vi "sort-sce-list.vi"(11 "模式列表":T1(array[cluster]) {"sce-pannel-list"."pannel"."ID" format="%02x"}) -> (3 "模式列表-sorted":T1(array[cluster]))   [LabVIEW 2019]
panel:
  in  "模式列表 4":T1(array[cluster]) {"sce-pannel-list"."pannel"."ID" format="%02x"}
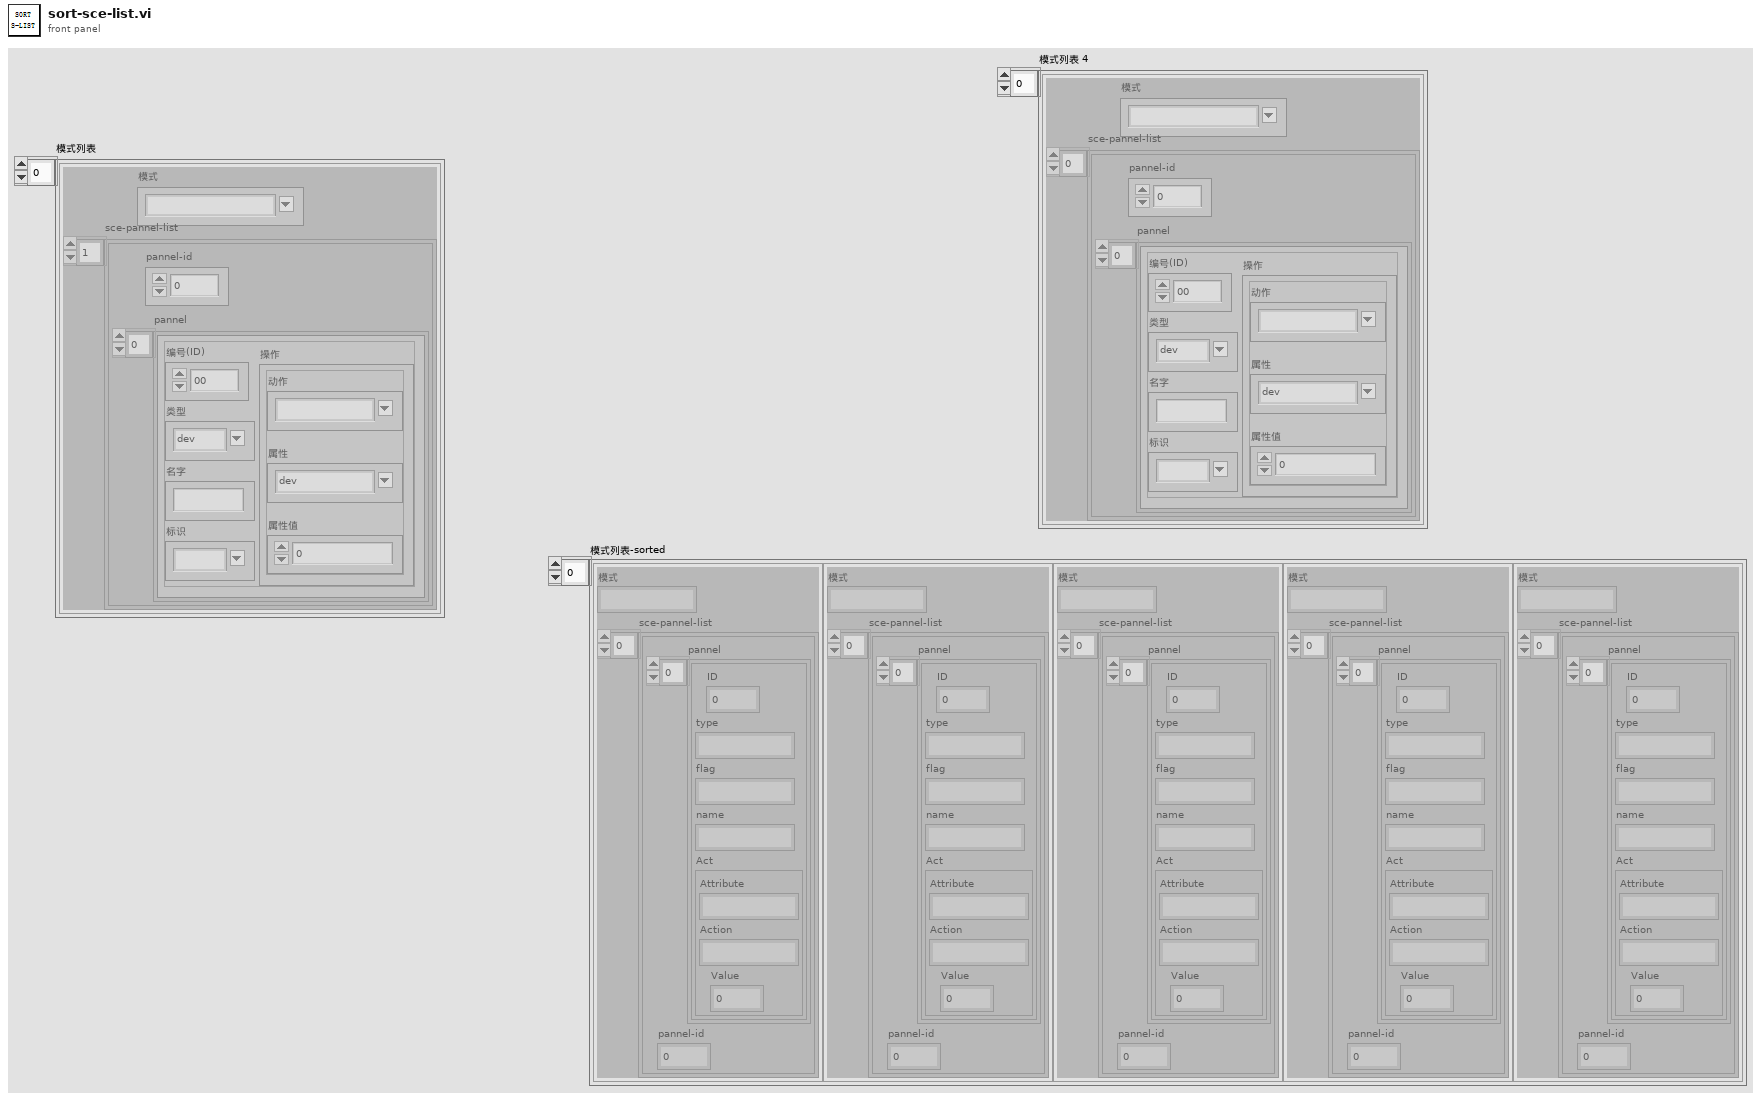
[diagram p1: front panel]
types:
  T1 = cluster{"模式":string, "sce-pannel-list":cluster{"pannel":cluster{"ID":u8, "type":string, "flag":string, "name":string, "Act":cluster{"Attribute":string, "Action":string, "Value":dbl}}[], "pannel-id":dbl}[]}[]
  T2 = cluster{"模式":string, "sce-pannel-list":cluster{"pannel":cluster{"ID":u8, "type":string, "flag":string, "name":string, "Act":cluster{"Attribute":string, "Action":string, "Value":dbl}}[], "pannel-id":dbl}[]}
  T3 = cluster{"pannel":cluster{"ID":u8, "type":string, "flag":string, "name":string, "Act":cluster{"Attribute":string, "Action":string, "Value":dbl}}[], "pannel-id":dbl}[]
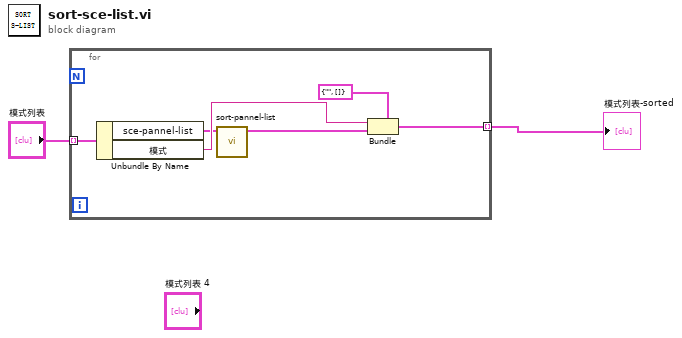
[diagram p0: block diagram]
diagram:
  n1 = for {
    tunnel: "模式列表" -> [w8] mode=indexing
    tunnel: [w5] -> w2 mode=indexing
    n2 = Unbundle By Name(w8) -> ("sce-pannel-list"=w4:T3, "模式"=w6:string)
    n3 = call "sort-pannel-list.vi"("sce-pannel-list"=w4) -> ("sorted-sce-pannel-list"=w3:T3)  [unwired: 10 in]
    n4 = Bundle(cluster=T2 {"模式"="", "sce-pannel-list"=[]} ("模式 2"), "模式"=w6, "sce-pannel-list"=w3) -> (w5:T2)
  }
  "模式列表-sorted" <- w2
